vi "Generate Data Frame Vectors.vi"(0 "RFFE RegWriteExt Command in":refnum<class "RFFE RegWriteExt Command.lvclass">, 11 "error in (no error)":errorcluster) -> (4 "RFFE RegWriteExt Command out":refnum<class "RFFE RegWriteExt Command.lvclass">, 6 "Data Frame Vectors":string[](array[string]), 15 "error out":errorcluster)   [LabVIEW 2018, in "MIPI RFFE API.lvlib" / "RFFE RegWriteExt Command.lvclass"]
uses:
  RFFE RegWriteExt Command.lvclass
  MIPI RFFE API.lvlib
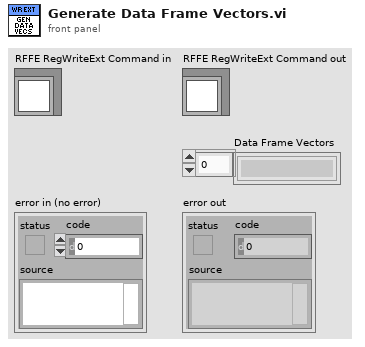
[diagram p1: front panel]
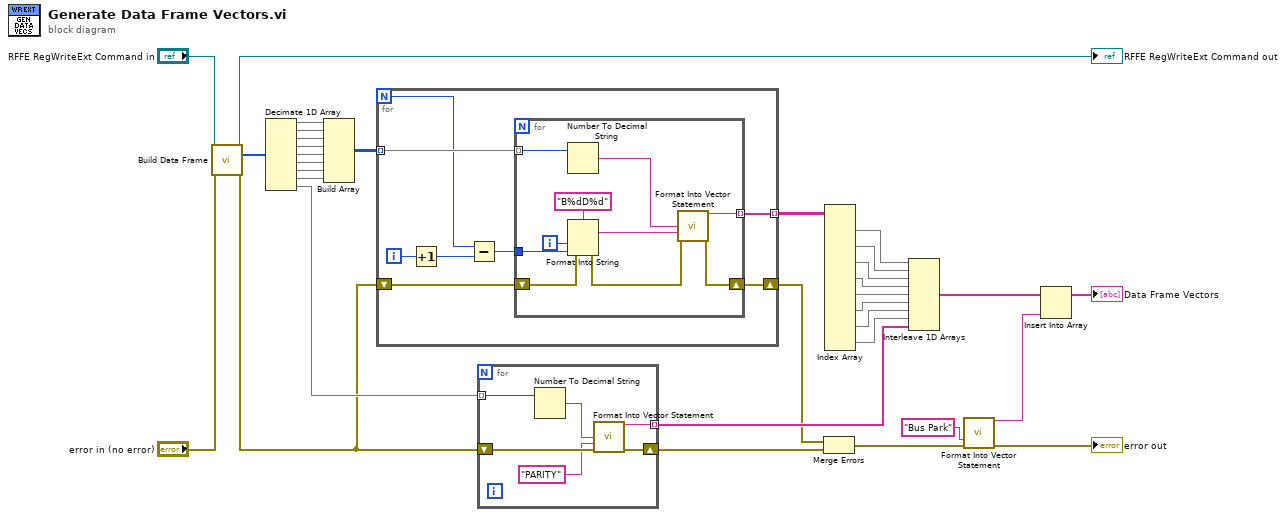
[diagram p0: block diagram]
diagram:
  n1 = call-dynamic "Build Data Frame.vi"("RFFE RegWriteExt Command in"="RFFE RegWriteExt Command in", "error in (no error)"="error in (no error)") -> ("RFFE RegWriteExt Command out"=→"RFFE RegWriteExt Command out":refnum<class "RFFE RegWriteExt Command.lvclass">, "Data Frame"=w31:u8[], "error out"=w7:errorcluster)  [unwired: 11 in]
  n2 = Decimate 1D Array(w31) -> (w30:u8[], w29:u8[], w28:u8[], w27:u8[], w26:u8[], w25:u8[], w24:u8[], w23:u8[], w12:u8[])
  n3 = Build Array(w30, w29, w28, w27, w26, w25, w24, w23) -> (w22:u8[][])
  n4 = for {
    N -> [w38]
    tunnel: w22 -> [w41] mode=indexing
    shift-right: [w39] -> w9
    shift-left: w7 -> [w40]
    tunnel: [w34] -> w21 mode=indexing
    i -> [w37]
    n5 = Increment(x=w37) -> (x+1=w36:i32)
    n6 = Subtract(x=w38, y=w36) -> (x-y=w35:i32)
    n7 = for {
      tunnel: w41 -> [w47] mode=indexing
      shift-right: [w43] -> w39
      shift-left: w40 -> [w48]
      tunnel: w35 -> [w49]
      tunnel: [w42] -> w34 mode=indexing
      i -> [w50]
      n8 = Number To Decimal String(number=w47) -> (decimal integer string=w46:string)  [unwired: 1 in]
      n9 = Format Into String(format string="B%dD%d", error in=w48, w50, w49) -> (resulting string=w45:string, error out=w44:errorcluster)  [unwired: 1 in]
      n10 = call "Format Into Vector Statement.vi"("DATA (0)"=w46, "Comment"=w45, "error in (no error)"=w44) -> ("Vector Statement"=w42:string, "error out"=w43:errorcluster)  [unwired: 11 in]
    }
  }
  n11 = for {
    shift-right: [w55] -> w10
    shift-left: w7 -> [w56]
    tunnel: w12 -> [w53] mode=indexing
    tunnel: [w52] -> w11 mode=indexing
    n12 = Number To Decimal String(number=w53) -> (decimal integer string=w57:string)  [unwired: 1 in]
    n13 = call "Format Into Vector Statement.vi"("DATA (0)"=w57, "Comment"="PARITY", "error in (no error)"=w56) -> ("Vector Statement"=w52:string, "error out"=w55:errorcluster)  [unwired: 11 in]
  }
  n14 = Merge Errors(w9, w10) -> (w3:errorcluster)
  n15 = Index Array(array=w21) -> (element #1=w20:string[], element #2=w19:string[], element #3=w18:string[], element #4=w17:string[], element #5=w16:string[], element #6=w15:string[], element #7=w14:string[], element #8=w13:string[])  [unwired: 16 in]
  n16 = Interleave 1D Arrays(w20, w19, w18, w17, w16, w15, w14, w13, w11) -> (w5:string[])
  n17 = call "Format Into Vector Statement.vi"("Comment"="Bus Park", "error in (no error)"=w3) -> ("Vector Statement"=w2:string, "error out"=→"error out":errorcluster)  [unwired: 12 in]
  n18 = Insert Into Array(array=w5, new element=w2) -> (→"Data Frame Vectors":string[])  [unwired: 1 in]
